vi "SaveScan_mk3.vi"(0 "Display Array":u16[][](array[numeric])=array125x512[64000 elements], 1 "Array":u16[][][](array[numeric]), 2 "selected path":path, 3 "Spec metadata":T6={"SPEC"={"CCD"={"ModuleNo"="HIS-Specim", "SerialNo"="V10E", "CCD Type"="iXon", "Counts"=0, "PixelNumber"=512, "PixelSize"=0.0, "Exposure(ms )"=10.0, "Average"=1, "Boxcar"=1, "binFactor"=1, "Reversion"=FALSE, "Andor"={"Temp. Target"=0, "Temp Stablized?"=FALSE, "Readout List"=[], "RreAmp List"=[], "VSS List"=[], "Readout"=4, "PreAmp"=0, "VSS"=0, "Temp. Min"=0, "Temp. Max"=0, "OutputAmp List"=[], "OutputAmp"=0}, "Kinetic No"=0, "AccumCT"=0.0, "KineticCT"=0.0, "AcqMode"=enum."Monitor", "SpectraProcess"=enum."Default", "Real AccumCT"=0.0, "Real KineticCT"=0.0, "Real Exposure"=0.0, "Ref"=[], "Graph"={"X "=[], "Y"=[]}, "Center to"=0.0, "Pulse"=0.0, "X Mode"=enum."Wavelength (nm)", "Background"=[], "Scan"=FALSE}, "SPEC Name"="", "User"={"COM"="", "GratingNo "=0, "Interval (ms )"=0, "Laser (nm)"=0.0}, "Gratings with PAT"=[], "ShutterID"=0, "Scanner4"={"Total Frames"=0, "Frames Dwell(s)"=0.0, "Z-Stack"=FALSE}, "SPEC Type"=""}, "i"=0}) -> ()   [LabVIEW 2016]
uses:
  Class/TIFF/TIFF ULS.lvclass
  Class/IFD/IFD.lvclass
  Class/Tag/IFD_Tag.lvclass/IFD_Tag.ctl
  Class/IFD/IFD.lvclass/IFD.ctl
  Class/TIFF/TIFF ULS.lvclass/TIFF ULS.ctl
  Class/IFD/Img Data Type.ctl
  Class/IFD/ULS/ULS Sigma Koki.vi
  Class/IFD/ULS/ULS PMT.vi
  Class/IFD/ULS/ULS Andor CCD.vi
  Class/IFD/Image Data/IFD RGB Image in.vi
  Class/IFD/IFD Add Tags.vi
  Class/Tag/Tag Create.vi
  Class/Tag/IFD_Tag.lvclass
panel:
  out "max value":u16
  in  "PMT Dwell(ms)":dbl
  in  "Scan Rate(sample/sec)":dbl=1000.0 format="%#_13g"
  in  "Objective":u32=1
  in  "Ref Img Array":u32[][](array[colorbox])
  in  "Ref img pixel size":dbl format="%#_13g"
  in  "input cluster":T1={"Name"="Specim", "Instrument"=enum."Spec", "ROI type"=enum."Rectangular", "X"={"X1"=0.1, "X2"=0.9}, "Y"={"Y1"=0.1, "Y2"=0.9}, "Pixel Size"=1.0}
  in  "ROI":cluster{"X1":sgl, "X2":sgl, "Y1":sgl, "Y2":sgl}={"X1"=0.0, "X2"=1.0, "Y1"=0.0, "Y2"=1.0}
  in  "Instrument":enum32{"OM", "PMT", "Spec"}(ring)=enum."Spec"
  in  "Stage Settings Array":T2(array[cluster])
  in  "Hardware Model":T3={"Controller"=enum."SHOT-304", "X Stage"="", "Y Stage"="", "Z Stage"="", "R Stage"=""}
  in  "Scan Dimension":T4={"ROI"=enum."Rectangle", "Z layer count"=255, "Time Lapse"=enum."None"}
  in  "Scanner Component":T5={"Detector"=enum."Andor CCD", "Mover"=enum."Sigmakoki Stage"}
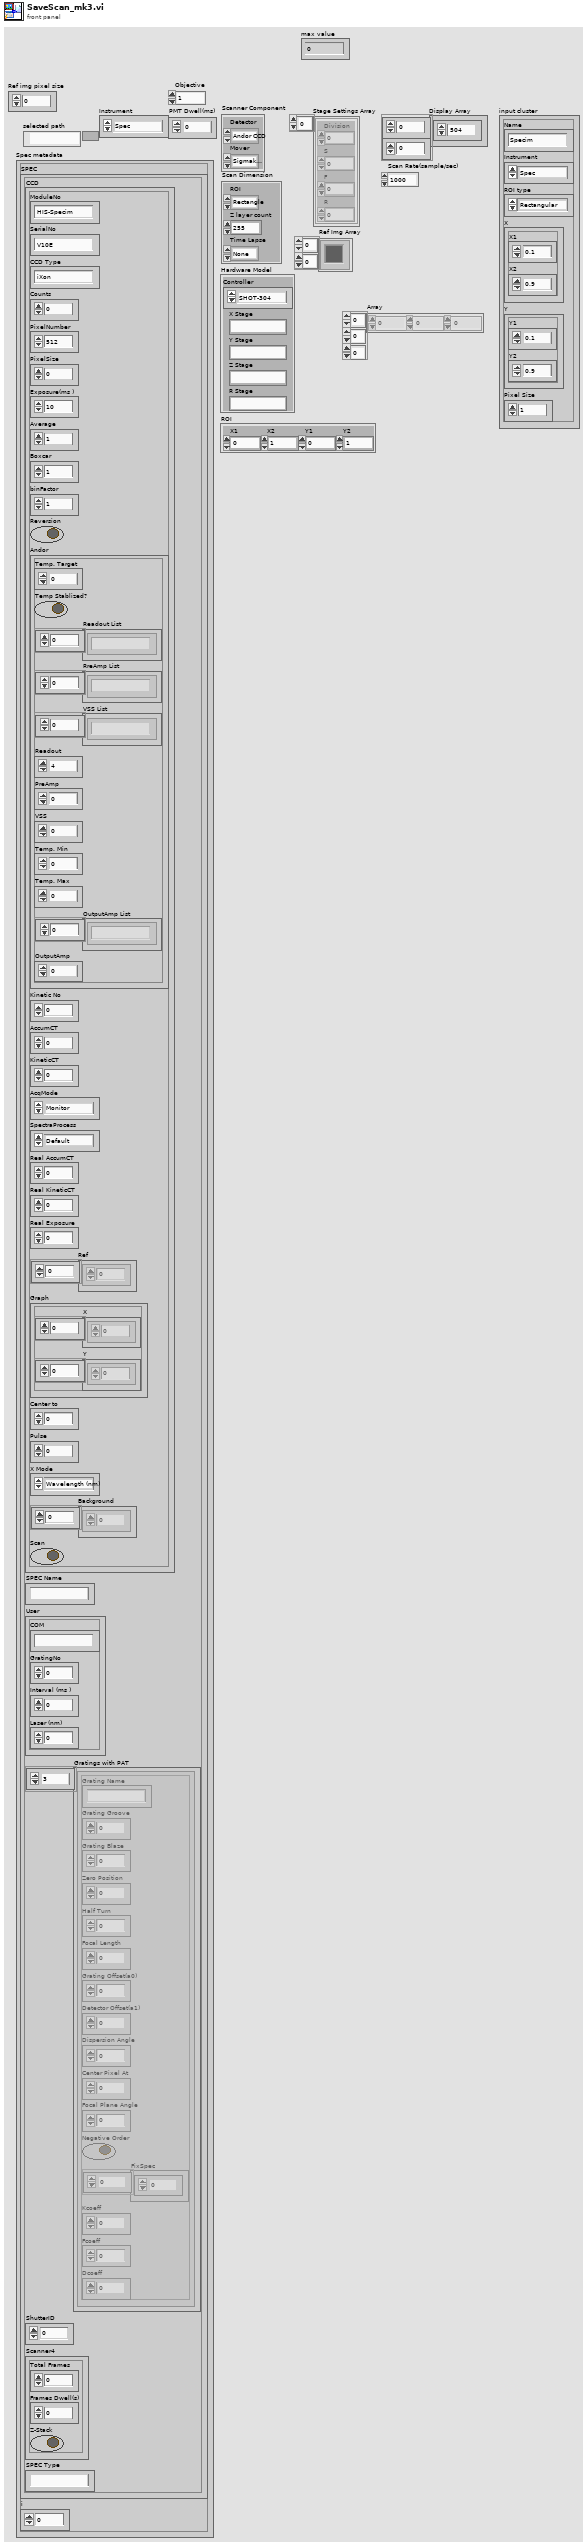
[diagram p1: front panel]
types:
  T1 = cluster{"Name":string, "Instrument":enum32{"OM", "PMT", "Spec"}, "ROI type":enum32{"View", "Dot", "Line", "Rectangular", "Square"}, "X":cluster{"X1":dbl, "X2":dbl}, "Y":cluster{"Y1":dbl, "Y2":dbl}, "Pixel Size":dbl}
  T2 = cluster{"Division":u8, "S":u32, "F":u32, "R":u32}[]
  T3 = cluster{"Controller":enum32{"GSC-01(PAT)", "SHOT-102", "SHOT-302", "SHOT-602", "SHOT-702", "FINE-503", "SHOT-204", "SHOT-304"}, "X Stage":string, "Y Stage":string, "Z Stage":string, "R Stage":string}
  T4 = cluster{"ROI":enum8{"Undefined: No Ref", "Point", "Line", "Rectangle", "Square"}, "Z layer count":u8, "Time Lapse":enum8{"None", "Toe to Head", "Head to Head"}}
  T5 = cluster{"Detector":enum16{"Mightex BUF CCD", "PMT", "Andor CCD"}, "Mover":enum16{"None", "Galvo", "Sigmakoki Stage"}}
  T6 = cluster{"SPEC":cluster{"CCD":cluster{"ModuleNo":string, "SerialNo":string, "CCD Type":string, "Counts":i32, "PixelNumber":i32, "PixelSize":dbl, "Exposure(ms )":dbl, "Average":i32, "Boxcar":i32, "binFactor":i32, "Reversion":bool, "Andor":cluster{"Temp. Target":i32, "Temp Stablized?":bool, "Readout List":string[], "RreAmp List":string[], "VSS List":string[], "Readout":u16, "PreAmp":u16, "VSS":u16, "Temp. Min":i32, "Temp. Max":i32, "OutputAmp List":string[], "OutputAmp":u16}, "Kinetic No":i32, "AccumCT":dbl, "KineticCT":dbl, "AcqMode":enum16{"Monitor", "Acquisition"}, "SpectraProcess":enum16{"Absorption", "TakeRef", "TakeBG", "Substraction", "Transmission", "ClearRef", "ClearBG", "Default"}, "Real AccumCT":dbl, "Real KineticCT":dbl, "Real Exposure":dbl, "Ref":sgl[], "Graph":cluster{"X ":sgl[], "Y":sgl[]}, "Center to":dbl, "Pulse":dbl, "X Mode":enum16{"Wavelength (nm)", "Pixel (um)", "Raman Shift (cm^-1)"}, "Background":sgl[], "Scan":bool}, "SPEC Name":string, "User":cluster{"COM":string, "GratingNo ":i32, "Interval (ms )":i32, "Laser (nm)":dbl}, "Gratings with PAT":cluster{"Grating Name":string, "Grating Groove":dbl, "Grating Blaze":dbl, "Zero Position":dbl, "Half Turn":dbl, "Focal Length":dbl, "Grating Offset(a0)":dbl, "Detector Offset(a1)":dbl, "Dispersion Angle":dbl, "Center Pixel At":dbl, "Focal Plane Angle":dbl, "Negative Order":bool, "FixSpec":dbl[], "Kcoeff":dbl, "Fcoeff":dbl, "Dcoeff":dbl}[], "ShutterID":i32, "Scanner4":cluster{"Total Frames":i32, "Frames Dwell(s)":dbl, "Z-Stack":bool}, "SPEC Type":string}, "i":u32}
  T7 = enum16{"open", "replace", "create", "open or create", "replace or create", "replace or create with confirmation"}
  T8 = cluster{"CCD Model Num":string, "Exposure time(ms)":sgl, "Average":u8, "Boxcar":u8, "Pixel Count":u32, "Readout Mode":enum8{"FVB", "Multi Track", "Random Track", "Single Track", "2D"}, "Spec Mode":enum8{"Wavelength(nm)", "Wavenumber(/cm)"}, "Grating Groove":u16, "Blaze":u16, "Data BG":enum8{"No BG", "Not Subtracted", "Subtracted"}, "Ref BG":enum8{"No BG", "Not Subtracted", "Subtracted"}, "Data Processed":enum8{"No Ref", "Not Processed", "Processed"}, "Process Method":enum8{"Not Selected", "Absorption", "Transmission", "Subtraction"}}
  T9 = enum8{"FVB", "Multi Track", "Random Track", "Single Track", "2D"}
  T10 = cluster{"X Value Array":sgl[], "Background Data":u16[], "Reference Data":u16[]}
  T11 = enum8{"Not Selected", "Absorption", "Transmission", "Subtraction"}
  T12 = enum16{"Undefined(DO NOT USE)", "pixel", "inch", "cm"}
  T13 = typedef "Img Data Type.ctl" = enum16{"U16", "RGB", "SGL"}
  T14 = enum16{"big-endian, network order", "native, host order", "little-endian"}
  T15 = enum16{"Wavelength (nm)", "Pixel (um)", "Raman Shift (cm^-1)"}
  T16 = cluster{"Grating Name":string, "Grating Groove":dbl, "Grating Blaze":dbl, "Zero Position":dbl, "Half Turn":dbl, "Focal Length":dbl, "Grating Offset(a0)":dbl, "Detector Offset(a1)":dbl, "Dispersion Angle":dbl, "Center Pixel At":dbl, "Focal Plane Angle":dbl, "Negative Order":bool, "FixSpec":dbl[], "Kcoeff":dbl, "Fcoeff":dbl, "Dcoeff":dbl}[]
  T17 = enum16{"Absorption", "TakeRef", "TakeBG", "Substraction", "Transmission", "ClearRef", "ClearBG", "Default"}
  T18 = cluster{"Grating Name":string, "Grating Groove":dbl, "Grating Blaze":dbl, "Zero Position":dbl, "Half Turn":dbl, "Focal Length":dbl, "Grating Offset(a0)":dbl, "Detector Offset(a1)":dbl, "Dispersion Angle":dbl, "Center Pixel At":dbl, "Focal Plane Angle":dbl, "Negative Order":bool, "FixSpec":dbl[], "Kcoeff":dbl, "Fcoeff":dbl, "Dcoeff":dbl}
  T19 = enum32{"View", "Dot", "Line", "Rectangular", "Square"}
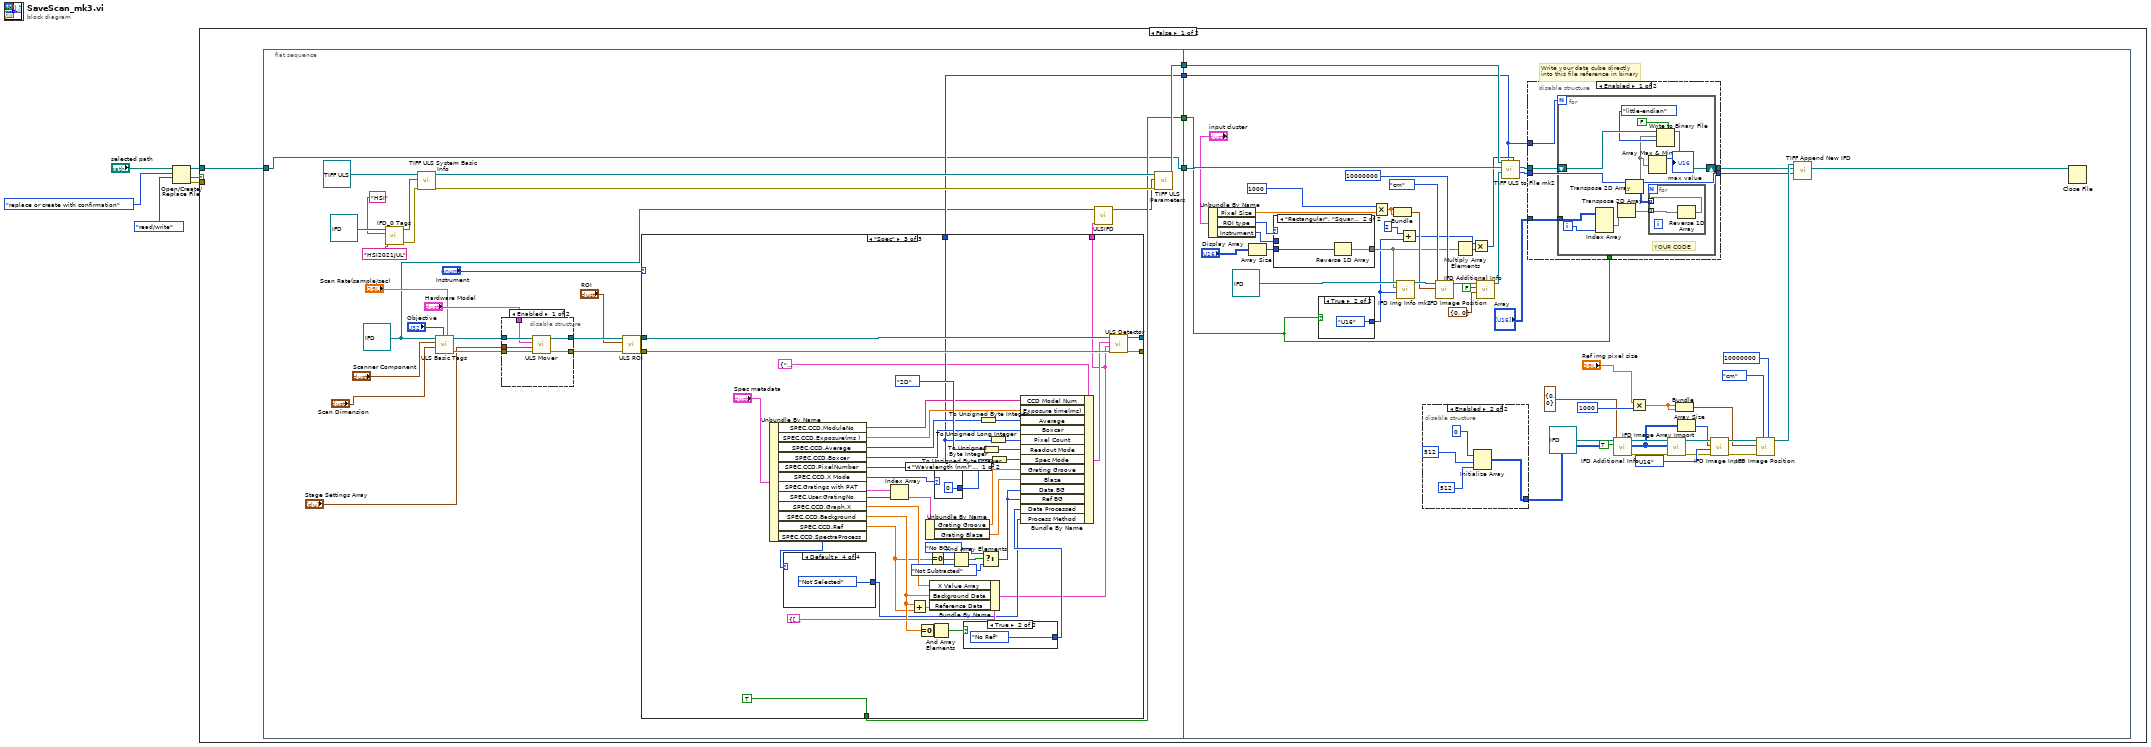
[diagram p0: block diagram]
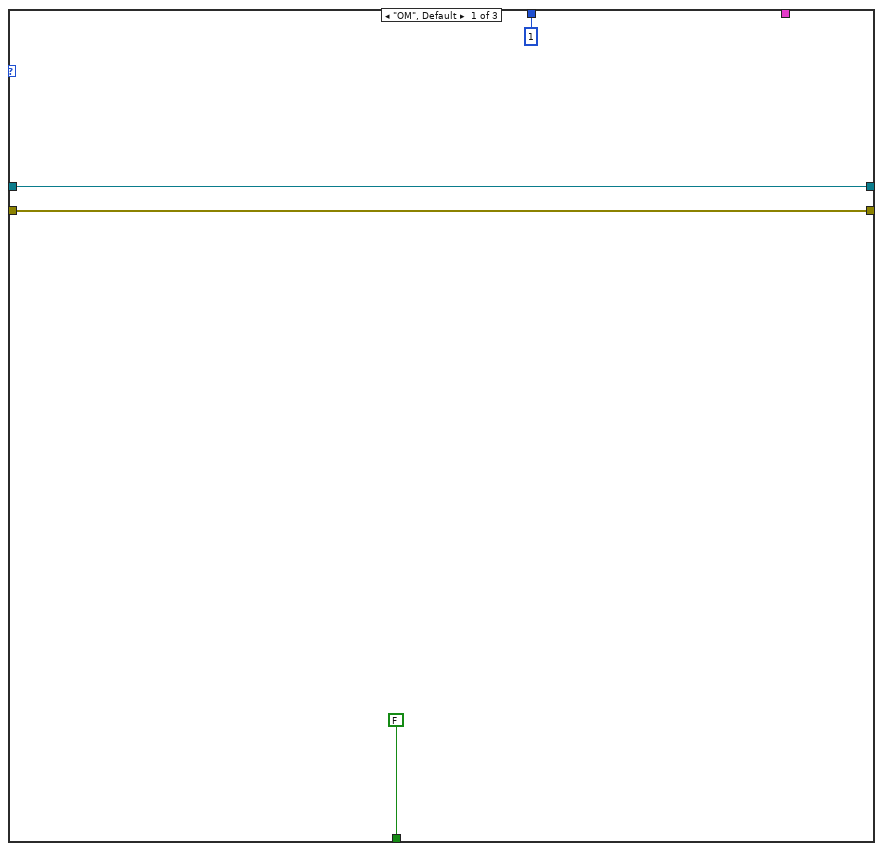
[diagram p3: hidden frame]
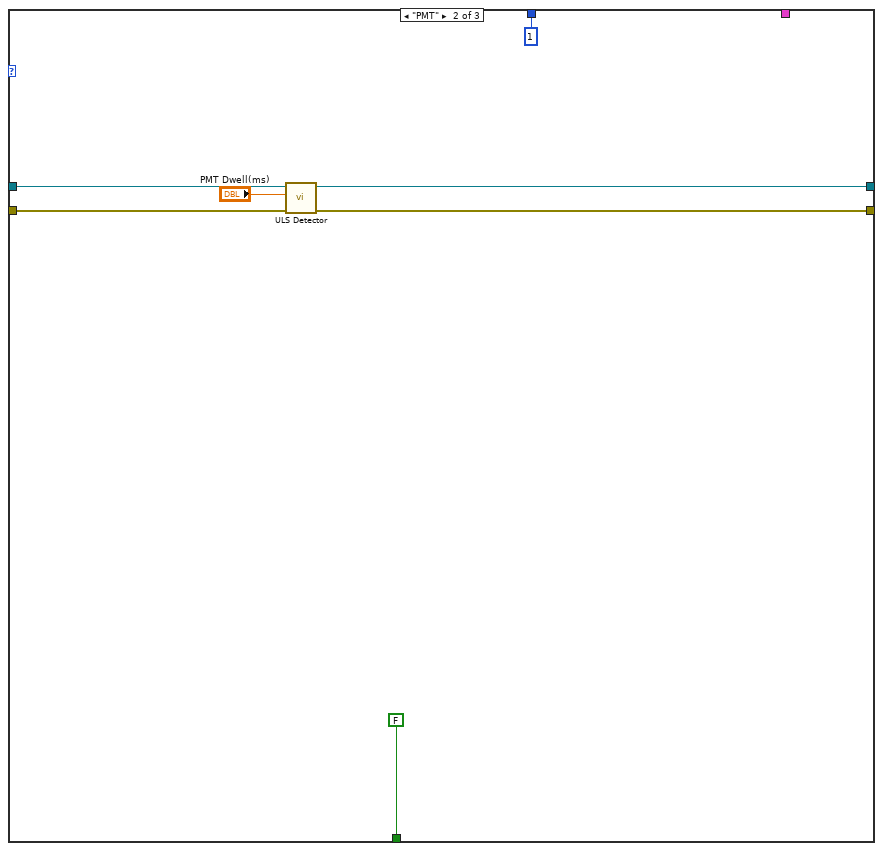
[diagram p4: hidden frame]
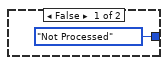
[diagram p5: hidden frame]
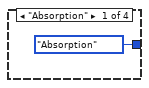
[diagram p6: hidden frame]
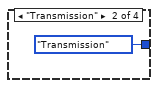
[diagram p7: hidden frame]
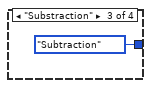
[diagram p8: hidden frame]
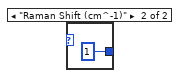
[diagram p9: hidden frame]
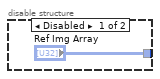
[diagram p10: hidden frame]
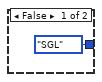
[diagram p12: hidden frame]
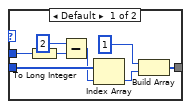
[diagram p13: hidden frame]
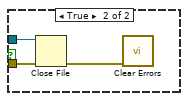
[diagram p14: hidden frame]
diagram:
  n1 = Open/Create/Replace File(file path (use dialog)="selected path", operation (0:open)=T7."replace or create with confirmation", access (0:read/write)=enum16{"read/write", "read-only", "write-only"}."read/write") -> (refnum out=w2:refnum<file>, cancelled=w3:bool, error out=w1:errorcluster)  [unwired: 3 in]
  n2 = case shown="False" w3 {
    tunnel: w2 -> [w11 w200]
    tunnel: w1 -> [_ w198]
    frame False {
      n3 = flat-sequence {
        tunnel: w11 -> [w23]
        tunnel: [w23] -> w10
        tunnel: [w31] -> w9
        tunnel: [w25] -> w8
        tunnel: [w24] -> w7
        tunnel: w10 -> [w151]
        tunnel: w9 -> [w150]
        tunnel: w8 -> [w109]
        tunnel: w7 -> [w115]
        frame #0 {
          w15 = refnum<class "IFD.lvclass"> refnum ("IFD in")
          n4 = call "IFD_0 Tags.vi"("Software Name and Version"="HSI2021JUL", "System Name"="HSI", "IFD in"=refnum<class "IFD.lvclass"> refnum) -> ("error out"=w27:errorcluster, "IFD out"=w39:refnum<class "IFD.lvclass">)  [unwired: 7 in]
          n5 = call "TIFF ULS System Basic Info.vi"("error in (no error)"=w27, "IFD"=w39, "TIFF in"=refnum<class "TIFF ULS.lvclass"> refnum ("TIFF ULS.lvclass")) -> ("error out"=w26:errorcluster, "TIFF out"=w32:refnum<class "TIFF ULS.lvclass">)  [unwired: 7 in]
          n6 = call "ULS Basic Tags.vi"("Scan Rate(sample/sec)"="Scan Rate(sample/sec)", "Objective"="Objective", "Scan Dimension"="Scan Dimension", "Scanner Component"="Scanner Component", "IFD in"=w15) -> ("error out"=w30:errorcluster, "IFD out"=w35:refnum<class "IFD.lvclass">)  [unwired: 5 in]
          n7 = disable-structure shown="Enabled" {
            disable-tunnel: w35 -> [w46 w48]
            disable-tunnel: [w45 w48] -> w34
            disable-tunnel: w30 -> [w44 w47]
            disable-tunnel: [w43 w47] -> w29
            disable-tunnel: "Hardware Model" -> [w42 _]
            disable-tunnel: "Stage Settings Array" -> [w41 _]
            frame Enabled {
              n8 = call-poly "ULS Mover.vi"("error in (no error)"=w44, "Settings Array"=w41, "Hardware Model"=w42, "IFD in"=w46) -> ("error out"=w43:errorcluster, "IFD out"=w45:refnum<class "IFD.lvclass">)  [unwired: 6 in]
            }
            frame Disabled {
            }
          }
          n9 = call "ULS ROI.vi"("error in (no error)"=w29, "ROI"="ROI", "IFD in"=w34) -> ("error out"=w28:errorcluster, "IFD out"=w33:refnum<class "IFD.lvclass">)  [unwired: 7 in]
          n10 = case shown="\"Spec\"" "Instrument" {
            tunnel: w33 -> [w52 w59 w100]
            tunnel: [w52 w58 w62] -> _
            tunnel: w28 -> [w51 w57 w82]
            tunnel: [w51 w56 w81] -> _
            tunnel: [1 ("PixelNumber") 1 ("PixelNumber") w80] -> w25
            tunnel: [FALSE FALSE TRUE] -> w24
            tunnel: [_ _ w60] -> w12
            frame "OM", Default {
            }
            frame "PMT" {
              n11 = call-poly "ULS Detector.vi"("error in (no error)"=w57, "Dwell(ms)"="PMT Dwell(ms)", "IFD in"=w59) -> ("error out"=w56:errorcluster, "IFD out"=w58:refnum<class "IFD.lvclass">)  [unwired: 7 in]
            }
            frame "Spec" {
              n12 = Unbundle By Name("Spec metadata") -> ("SPEC.CCD.ModuleNo"=w83:string, "SPEC.CCD.Exposure(ms )"=w84:dbl, "SPEC.CCD.Average"=w85:i32, "SPEC.CCD.Boxcar"=w86:i32, "SPEC.CCD.PixelNumber"=w80:i32, "SPEC.CCD.X Mode"=w88:T15, "SPEC.Gratings with PAT"=w89:T16, "SPEC.User.GratingNo"=w90:i32, "SPEC.CCD.Graph.X"=w95:sgl[], "SPEC.CCD.Background"=w77:sgl[], "SPEC.CCD.Ref"=w76:sgl[], "SPEC.CCD.SpectraProcess"=w96:T17)
              n13 = case shown="Default" w96 {
                tunnel: [T11."Absorption" ("Process Method") T11."Transmission" ("Process Method") T11."Subtraction" ("Process Method") T11."Not Selected" ("Process Method")] -> w69
                frame "Absorption" {
                }
                frame "Transmission" {
                }
                frame "Substraction" {
                }
                frame Default {
                }
              }
              n14 = Index Array(array=w89, index=w90) -> (element=w91:T18)
              n15 = Add(x=w77, y=w76) -> (x+y=w75:sgl[])
              n16 = Equal To 0?(x=w77) -> (x = 0?=w99:bool[])
              n17 = Unbundle By Name(w91) -> ("Grating Groove"=w92:dbl, "Grating Blaze"=w93:dbl)
              n18 = Equal To 0?(x=w76) -> (x = 0?=w97:bool[])
              n19 = Bundle By Name(cluster=T10 {"X Value Array"=[], "Background Data"=[], "Reference Data"=[]} ("Array Data"), "X Value Array"=w95, "Background Data"=w77, "Reference Data"=w75) -> (w60:T10)
              n20 = And Array Elements(Boolean array=w99) -> (logical AND=w71:bool)
              n21 = case shown="\"Wavelength (nm)\", Default" w88 {
                tunnel: [u8 0 u8 1] -> w65
                frame "Wavelength (nm)", Default {
                }
                frame "Raman Shift (cm^-1)" {
                }
              }
              n22 = And Array Elements(Boolean array=w97) -> (logical AND=w98:bool)
              n23 = case shown="True" w71 {
                tunnel: [enum8{"No Ref", "Not Processed", "Processed"}."Not Processed" ("Data Processed") enum8{"No Ref", "Not Processed", "Processed"}."No Ref" ("Data Processed")] -> w70
                frame False {
                }
                frame True {
                }
              }
              n24 = To Unsigned Byte Integer(number=w85) -> (unsigned 8bit integer=w67:u8)
              n25 = Select(t=enum8{"No BG", "Not Subtracted", "Subtracted"}."No BG" ("Data BG"), s=w98, f=enum8{"No BG", "Not Subtracted", "Subtracted"}."Not Subtracted") -> (s? t:f=w72:enum8{"No BG", "Not Subtracted", "Subtracted"})
              n26 = To Unsigned Byte Integer(number=T9."2D" ("Readout Mode")) -> (unsigned 8bit integer=w66:u8)
              n27 = To Unsigned Long Integer(number=w80) -> (unsigned 32bit integer=w63:u32)
              n28 = To Unsigned Byte Integer(number=w65) -> (unsigned 8bit integer=w64:u8)
              n29 = Bundle By Name(cluster=T8 {"CCD Model Num"="", "Exposure time(ms)"=0.0, "Average"=1, "Boxcar"=0, "Pixel Count"=1, "Readout Mode"=enum."FVB", "Spec Mode"=enum."Wavelength(nm)", "Grating Groove"=1200, "Blaze"=500, "Data BG"=enum."No BG", "Ref BG"=enum."No BG", "Data Processed"=enum."No Ref", "Process Method"=enum."Not Selected"} ("General Info"), "CCD Model Num"=w83, "Exposure time(ms)"=w84, "Average"=w67, "Boxcar"=w86, "Pixel Count"=w63, "Readout Mode"=w66, "Spec Mode"=w64, "Grating Groove"=w92, "Blaze"=w93, "Data BG"=w72, "Ref BG"=w72, "Data Processed"=w70, "Process Method"=w69) -> (w61:T8)
              n30 = call-poly "ULS Detector.vi"("error in (no error)"=w82, "Array Data"=w60, "General Info"=w61, "IFD in"=w100) -> ("error out"=w81:errorcluster, "IFD out"=w62:refnum<class "IFD.lvclass">)  [unwired: 6 in]
            }
          }
          n31 = call "ULSIFD.vi"("IFD in"=w15, "Array Data"=w12) -> ("IFD out"=w16:refnum<class "IFD.lvclass">)  [unwired: 7 in]
          n32 = call "TIFF ULS Parameters.vi"("error in (no error)"=w26, "IFD"=w16, "TIFF in"=w32) -> ("TIFF out"=w31:refnum<class "TIFF ULS.lvclass">)  [unwired: 7 in, 1 out]
        }
        frame #1 {
          # "Write your data cube directly\ninto this file reference in binary"
          n33 = Unbundle By Name("input cluster") -> ("Pixel Size"=w147:dbl, "ROI type"=w126:T19, "Instrument"=w125:enum32{"OM", "PMT", "Spec"})
          n34 = Array Size(array="Display Array") -> (size(s)=w146:i32[])
          n35 = case shown="\"Rectangular\", \"Square\"" w126 {
            tunnel: w146 -> [w195 w197]
            tunnel: [w192 w196] -> w145
            tunnel: w125 -> [w191 _]
            frame Default {
              n36 = To Long Integer(number=w191) -> (32bit integer=w188:i32)
              n37 = Subtract(x=2, y=w188) -> (x-y=w190:i32)
              n38 = Index Array(array=w195, index=w190) -> (element=w194:i32)
              n39 = Build Array(1, w194) -> (w192:i32[])
            }
            frame "Rectangular", "Square" {
              n40 = Reverse 1D Array(array=w197) -> (reversed array=w196:i32[])
            }
          }
          n41 = case shown="True" w115 {
            tunnel: [Img_Data_Type."SGL" ("Data type") Img_Data_Type."U16" ("Data type")] -> w124
            frame False {
            }
            frame True {
            }
          }
          n42 = Multiply(x=1000, y=w147) -> (x*y=w155:dbl)
          n43 = Bundle(w155, w155) -> (w154:cluster{dbl, dbl})  [unwired: 1 in]
          n44 = call "IFD Img Info mk2.vi"("Data type"=w124, "size(s)"=w145, "IFD in"=refnum<class "IFD.lvclass"> refnum) -> ("IFD out"=w157:refnum<class "IFD.lvclass">)  [unwired: 7 in, 1 out]
          n45 = Add(x=2, y=w124) -> (x+y=w122:i32)
          n46 = disable-structure shown="Enabled" {
            disable-tunnel: ["Ref Img Array" w162] -> w110
            frame Disabled {
            }
            frame Enabled {
              n47 = Initialize Array(u16 0 ("element"), 512 ("dimension size"), 512 ("dimension size")) -> (w162:u16[][])
            }
          }
          n48 = call "IFD Image Position.vi"("Public Denominator"=u32 10000000, "Basic Unit"=T12."cm", "Pixel Size"=w154, "IFD in"=w157) -> ("IFD out"=w159:refnum<class "IFD.lvclass">)  [unwired: 6 in, 1 out]
          n49 = Multiply Array Elements(1:w145) -> (0:w144:i32)
          n50 = Multiply(x=w122, y=w144) -> (x*y=w143:i32)
          n51 = call "IFD Additional Info.vi"("Page"=cluster{"Total Pages":u16, "Current Page":u16} {"Total Pages"=0, "Current Page"=0}, "Is ref?"=FALSE, "IFD in"=w159) -> ("IFD out"=w149:refnum<class "IFD.lvclass">)  [unwired: 7 in, 1 out]
          n52 = call "TIFF ULS to File mk2.vi"("Image Size"=w143, "Layer Count"=w109, "Basic IFD"=w149, "refnum in"=w151, "TIFF ULS in"=w150) -> ("Reference Offset"=w118:u32, "refnum out"=w119:refnum<file>)  [unwired: 4 in, 1 out]
          n53 = disable-structure shown="Enabled" {
            disable-tunnel: w119 -> [w170 w185]
            disable-tunnel: w118 -> [w168 w184]
            disable-tunnel: [w169 w185] -> w117
            disable-tunnel: [w168 w184] -> w116
            disable-tunnel: w115 -> [_ _]
            disable-tunnel: "Array" -> [w167 _]
            disable-tunnel: w109 -> [w166 _]
            frame Enabled {
              n54 = for {
                N: w166 -> [_]
                tunnel: w167 -> [w179]
                shift-right: [w180] -> w169
                shift-left: w170 -> [w181]
                i -> [w177]
                # "YOUR CODE"
                n55 = Index Array(array=w179, index (dim 2)=w177) -> (element=w176:u16[][])  [unwired: 2 in]
                n56 = Transpose 2D Array(2D array=w176) -> (transposed array=w174:u16[][])
                n57 = for {
                  tunnel: w174 -> [w183] mode=indexing
                  tunnel: [w182] -> w175 mode=indexing
                  n58 = Reverse 1D Array(array=w183) -> (reversed array=w182:u16[])
                }
                n59 = Transpose 2D Array(2D array=w175) -> (transposed array=w172:u16[][])
                n60 = Array Max & Min(array=w172) -> (max value=→"max value":u16)  [unwired: 3 out]
                n61 = Write to Binary File(file (use dialog)=w181, data=w172, 5:FALSE ("prepend array or string size? (T)"), 9:T14."little-endian" ("byte order (0:big-endian, network order)")) -> (refnum out=w180:refnum<file>)  [unwired: 2 in, 2 out]
              }
            }
            frame Disabled {
            }
          }
          n62 = call "IFD Additional Info.vi"("Page"=cluster{"Total Pages":u16, "Current Page":u16} {"Total Pages"=0, "Current Page"=0}, "Is ref?"=TRUE, "IFD in"=refnum<class "IFD.lvclass"> refnum) -> ("error out"=w130:errorcluster, "IFD out"=w140:refnum<class "IFD.lvclass">)  [unwired: 7 in]
          n63 = Multiply(x="Ref img pixel size", y=1000) -> (x*y=w134:dbl)
          n64 = call-poly "IFD Image Array Import.vi"("error in (no error)"=w130, "RGB Array"=w110, "IFD in"=w140) -> ("error out"=w129:errorcluster, "IFD out"=w139:refnum<class "IFD.lvclass">)  [unwired: 7 in]
          n65 = Bundle(w134, w134) -> (w133:cluster{dbl, dbl})  [unwired: 1 in]
          n66 = Array Size(array=w110) -> (size(s)=w113:i32[])
          n67 = call "IFD Image Input.vi"("error in (no error)"=w129, "Data type"=Img_Data_Type."U16", "size(s)"=w113, "IFD in"=w139) -> ("error out"=w128:errorcluster, "IFD out"=w137:refnum<class "IFD.lvclass">)  [unwired: 6 in]
          n68 = call "IFD Image Position.vi"("Public Denominator"=u32 10000000, "Basic Unit"=T12."cm", "error in (no error)"=w128, "Pixel Size"=w133, "IFD in"=w137) -> ("IFD out"=w127:refnum<class "IFD.lvclass">)  [unwired: 5 in, 1 out]
          n69 = call "TIFF Append New IFD.vi"("Last Reference Offset"=w116, "refnum in"=w117, "IFD in"=w127) -> ("refnum out"=w112:refnum<file>)  [unwired: 7 in, 1 out]
          n70 = Close File(refnum=w112) -> ()  [unwired: 1 in, 2 out]
        }
      }
    }
    frame True {
      n71 = Close File(refnum=w200, error in=w198) -> (error out=w199:errorcluster)  [unwired: 1 out]
      n72 = call <vilib>:"Clear Errors.vi"("error in (no error)"=w199) -> ()  [unwired: 5 in, 2 out]
    }
  }
